vi "Post-Project-Copying Process - Stage 1.vi"(6 "Debug":bool, 8 "error in":errorcluster, 11 "PluginGenerator_MetaDataObj":refnum<class "PluginGenerator_MetaDataObj.lvclass">) -> (0 "error out":errorcluster, 3 "PluginGenerator_MetaDataObj out":refnum<class "PluginGenerator_MetaDataObj.lvclass">, 4 "Result for debugging":cluster{"Name":string, picture[]}[](array[cluster]))   [LabVIEW 2023, in "Plugin Generator.lvlib"]
uses:
  Plugin Generator.lvlib
  PluginGenerator_MetaDataObj/PluginGenerator_MetaDataObj.lvclass
  c:/perforce/build/exports/ni/nito/nitoolchainlabview2023eng64/official/export/23.3/23.3.0f52/win/resource/dialog/NewProjectWizard/MetaDataObj/MetaDataObj.lvclass
  <resource>/dialog/NewProjectWizard/MetaDataObj/MetaDataObj.lvclass/MetaDataObj.ctl
  PluginGenerator_MetaDataObj/Accessors/Read User Project Path.vi
  <resource>/dialog/NewProjectWizard/MetaDataObj/Accessors/Read Project Name.vi
  <resource>/dialog/NewProjectWizard/MetaDataObj/Accessors/Read Overlay Pixmap.vi
  Icon/Apply Icon into VIs.vi
  Generate gRPC relevant name.vi
  <resource>/dialog/NewProjectWizard/MetaDataObj/Accessors/Read Project Root.vi
  <vilib>/dlg_ctls.llb/Space Constant.vi
  <resource>/dialog/NewProjectWizard/MetaDataObj/Accessors/Read Project Path.vi
  Icon/Change Icon Text to Project Name.vi
  Project Item Recursion.vi
  <vilib>/LabVIEW Icon API/Get VI Icon.vi
  <vilib>/LabVIEW Icon API/Support/Get Data from Icon Class.vi
  <vilib>/LabVIEW Icon API/lv_icon/Classes/Layer/Substitute Layer.vi
  <vilib>/LabVIEW Icon API/Support/Get Icon Class from Data.vi
  <vilib>/LabVIEW Icon API/Set VI Icon.vi
  <vilib>/LabVIEW Icon API/Get Flattened Image.vi
  <vilib>/picture/picture.llb/Draw Flattened Pixmap.vi
  <vilib>/LabVIEW Icon API/Set Text Icon/Set Icon.vi
  <vilib>/Utility/EditLVLibs/Rename And Move Entire Library By Name.vi
  <vilib>/Utility/EditLVLibs/Rename And Move Entire Library By Path.vi
  <vilib>/LabVIEW Icon API/lv_icon/Classes/Icon/Icon.lvclass
  <vilib>/Utility/EditLVProj/Edit LVProj.lvlib
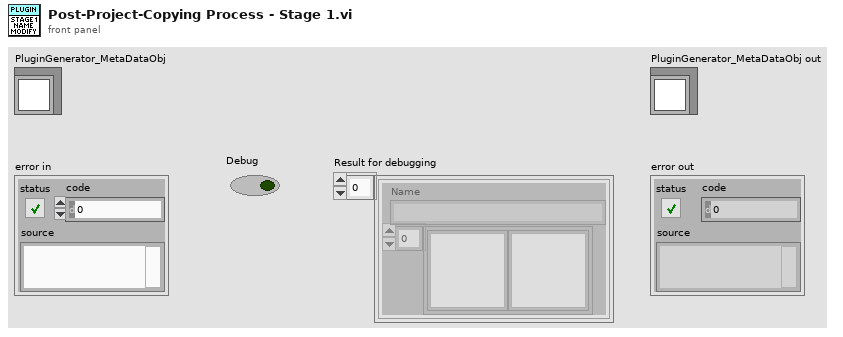
[diagram p1: front panel]
types:
  T1 = typedef "Plugin Generator.lvlib/Plugin OS.ctl" = enum16{"Linux RT", "Env Server"}
  T2 = typedef "Edit LVProj.lvlib/Library And VI References.ctl" = cluster{"Target Reference":refnum<vi>, "VI References":refnum<vi>[], "Library References":refnum<vi>[]}
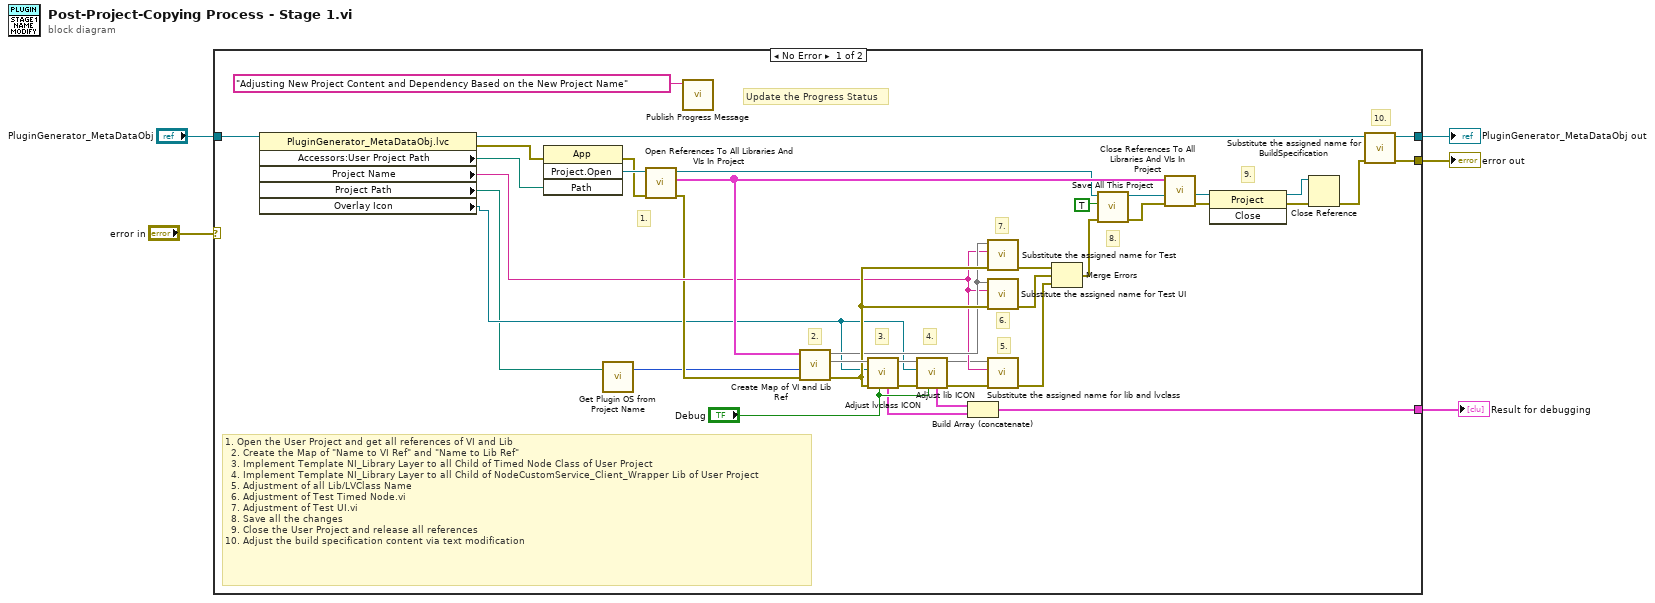
[diagram p0: block diagram]
diagram:
  n1 = case shown="No Error" "error in" {
    selector: "error in" -> [_ w44]
    tunnel: [w12 _] -> w5
    tunnel: "PluginGenerator_MetaDataObj" -> [w32 w45]
    tunnel: [w20 w45] -> w3
    tunnel: [w19 w44] -> w2
    frame No Error {
      # "10."
      # "Update the Progress Status"
      # "9."
      # "2."
      # "8."
      # "7."
      # "6."
      # "5."
      # "4."
      # "3."
      # "1."
      # "1. Open the User Project and get all references of VI and Lib\n  2. Create the Map of \"Name to VI Ref\" and \"Name to Lib Ref\"\n  3. Implement Template NI_Library Layer to all Child of Timed Node Class of User Project\n  4. Implement Template NI_Library Layer to all Child of NodeCustomService_Client_Wrapper Lib of User Project\n  5. Adjustment of all Lib/LVClass Name\n  6. Adjustment of Test Timed Node.vi\n  7. Adjustment of Test UI.vi\n  8. Save all the changes\n  9. Close the User Project and release all references\n10. Adjust the build specification content via text modification"
      n2 = property class="PluginGenerator_MetaDataObj.lvc"(reference=w32) -> (reference out=w21:refnum<class "PluginGenerator_MetaDataObj.lvclass">, error out=w24:errorcluster, "Accessors:User Project Path"=w10:path, "Project Name"=w22:string, "Project Path"=w7:path, "Overlay Icon"=w8:refnum<class "Icon.lvclass">)  [unwired: 1 in]
      n3 = invoke class="App" method="Project.Open"(error in=w24, "Path"=w10) -> (error out=w23:errorcluster, "Project:Open"=w31:refnum<vi>)  [unwired: 2 in, 2 out]
      n4 = call "Get Plugin OS from Project Name.vi"("Project Path"=w7) -> ("Plugin OS"=w6:T1)  [unwired: 2 in]
      n5 = call <vilib>:"Open References To All Libraries And VIs In Project.vi"("error in (no error)"=w23, "Project in"=w31) -> ("error out"=w9:errorcluster, "VI and Library References"=w42:T2[], "Project out"=w40:refnum<vi>)  [unwired: 7 in]
      n6 = call "Publish Progress Message.vi"("Progress"="Adjusting New Project Content and Dependency Based on the New Project Name") -> ()  [unwired: 11 in]
      n7 = call "Create Map of VI and Lib Ref.vi"("error in"=w9, "Plugin OS"=w6, "VI and Library References"=w42) -> ("error out"=w35:errorcluster, "Map - LibRef"=w38:map{string, refnum<vi>}, "Map - VIRef"=w34:map{string, refnum<vi>})  [unwired: 6 in]
      n8 = call "Adjust lvclass ICON.vi"("Debug"="Debug", "error in"=w35, "Overlay Icon"=w8, "Name to Lib Map"=w38) -> ("error out"=w16:errorcluster, "Name to Lib Map out"=w18:map{string, refnum<vi>}, "Result for debugging"=w13:cluster{"Name":string, picture[]}[])  [unwired: 5 in]
      n9 = call "Adjust lib ICON.vi"("Debug"="Debug", "error in"=w16, "Overlay Icon"=w8, "Name to Lib Map"=w18) -> ("error out"=w11:errorcluster, "Name to Lib Map out"=w17:map{string, refnum<vi>}, "Result for debugging"=w14:cluster{"Name":string, picture[]}[])  [unwired: 5 in]
      n10 = Build Array (concatenate)(w14, w13) -> (w12:cluster{"Name":string, picture[]}[])
      n11 = call "Substitute the assigned name for Test.vi"("error in"=w35, "Project Name"=w22, "Name to VI Map"=w34) -> ("error out"=w43:errorcluster)  [unwired: 8 in]
      n12 = call "Substitute the assigned name for Test UI.vi"("error in"=w35, "Project Name"=w22, "Name to VI Map"=w34) -> ("error out"=w37:errorcluster)  [unwired: 8 in]
      n13 = call "Substitute the assigned name for lib and lvclass.vi"("error in"=w11, "Project Name"=w22, "Name to Lib Map"=w17) -> ("error out"=w36:errorcluster)  [unwired: 7 in, 1 out]
      n14 = Merge Errors(w43, w37, w36) -> (w33:errorcluster)
      n15 = call <vilib>:"Save All This Project.vi"("error in (no error)"=w33, "Exclude Dependencies? (F)"=TRUE, "Project in"=w40) -> ("error out"=w39:errorcluster, "Project out"=w28:refnum<vi>)  [unwired: 7 in]
      n16 = call <vilib>:"Close References To All Libraries And VIs In Project.vi"("error in (no error)"=w39, "VI and Library References"=w42) -> ("error out"=w27:errorcluster)  [unwired: 9 in]
      n17 = invoke class="Project" method="Close"(reference=w28, error in=w27) -> (reference out=w29:refnum<vi>, error out=w30:errorcluster)  [unwired: 1 in, 1 out]
      n18 = Close Reference(reference=w29, error in (no error)=w30) -> (error out=w26:errorcluster)
      n19 = call "Substitute the assigned name for BuildSpecification.vi"("error in"=w26, "PluginGenerator_MetaDataObj"=w21) -> ("error out"=w19:errorcluster, "PluginGenerator_MetaDataObj out"=w20:refnum<class "PluginGenerator_MetaDataObj.lvclass">)  [unwired: 8 in]
    }
    frame Error {
    }
  }
  "error out" <- w2
  "Result for debugging" <- w5
  "PluginGenerator_MetaDataObj out" <- w3
